vi "0-Do Overlays.vi"(0 "Image Reference\nand Descriptor":cluster{"Image Out":T2, "Image Descriptor":T3} {"Image Descriptor"."Upper-Left Corner Coordinates"."North" format="%#_10f"; "Image Descriptor"."Upper-Left Corner Coordinates"."East" format="%#_8f"}, 1 "Missions":refnum<class "GenericMission.lvclass">[](array[class]), 2 "No Sail Circles":T1[](array[typedef]), 5 "Waypoints":T8, 7 "Current Waypoint #":T7, 9 "Heading":T5 format="%05.1f", 11 "Sail Position":T6=0.5, 12 "Robot UTM Location":T4 {"North" format="%#_10f"; "East" format="%#_8f"}) -> (4 "Image out":T2)   [LabVIEW 2011]
doc: "Overlays waypoints and a boat icon on the image."
uses:
  <vilib>/vision/Image Controls.llb/IMAQ Image.ctl
  0x2-OCU-Think Comm/0x2 Typedefs/Waypoints List.ctl
  2-Think/2 Classes/Waypoint/Waypoint.lvclass
  0x2-OCU-Think Comm/0x2 Typedefs/Current Waypoint.ctl
  2-Think/2 Typedefs/sail setpt.ctl
  2-Think/2 Typedefs/heading.ctl
  2-Think/2 Typedefs/UTM Location.ctl
  0-Image Descriptor.ctl
  2-Think/2 Classes/Missions/GenericMission/GenericMission.lvclass
  2-Think/2 Typedefs/UTM Circle.ctl
panel:
  out "Boat Outside Img":bool
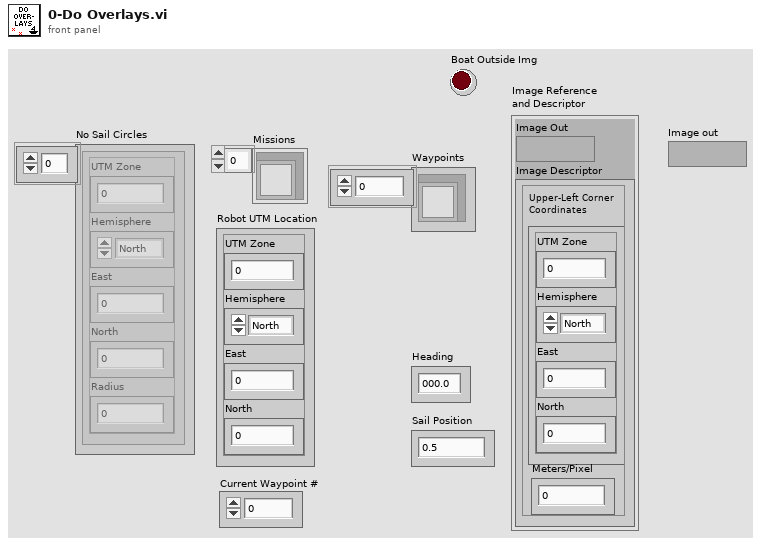
[diagram p1: front panel]
types:
  T1 = typedef "UTM Circle.ctl" = cluster{"UTM Zone":dbl, "Hemisphere":enum16{"North", "South"}, "East":dbl, "North":dbl, "Radius":dbl}
  T2 = typedef "IMAQ Image.ctl" = refnum<image>
  T3 = typedef "0-Image Descriptor.ctl" = cluster{"Upper-Left Corner Coordinates":T4, "Meters/Pixel":dbl}
  T4 = typedef "UTM Location.ctl" = cluster{"UTM Zone":dbl, "Hemisphere":enum16{"North", "South"}, "East":dbl, "North":dbl}
  T5 = typedef "heading.ctl" = dbl
  T6 = typedef "sail setpt.ctl" = dbl
  T7 = typedef "Current Waypoint.ctl" = i32
  T8 = typedef "Waypoints List.ctl" = refnum<class "Waypoint.lvclass">[]
  T9 = typedef "Overlay References.ctl" = cluster{"Boat Icon, Unroatated":T2, "Boat Icon, Rotated":T2, "Sail Icon, Unrotated":T2, "Sail Icon, Rotated":T2}
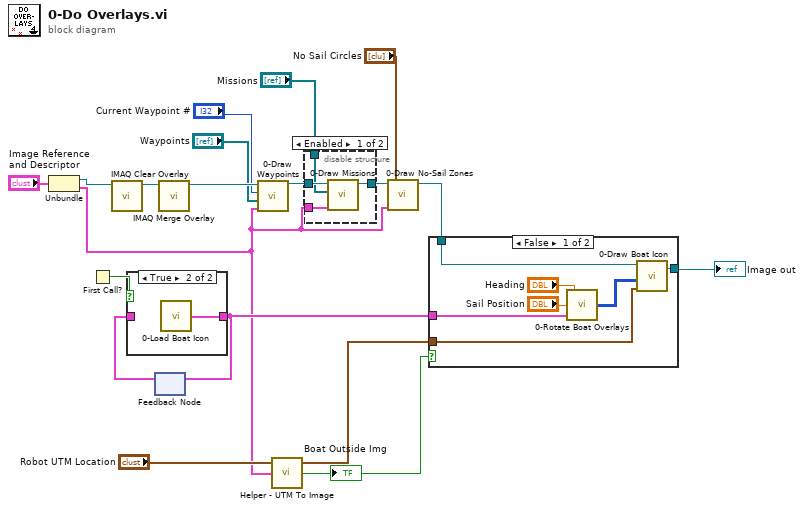
[diagram p0: block diagram]
diagram:
  n1 = Unbundle("Image Reference\nand Descriptor") -> ("Image Out"=w7:T2, "Image Descriptor"=w4:T3)
  n2 = First Call?() -> (First Call?: T/F=w16:bool)
  n3 = call "IMAQ Clear Overlay"("Image"=w7) -> ("Image Out"=w19:T2)  [unwired: 2 in, 8 out]
  n4 = feedback #1() -> (w14:T9)  [unwired: 1 in]
  n5 = case shown="True" w16 {
    tunnel: [w20 w21] -> w15
    tunnel: w14 -> [w20 _]
    frame False {
      # "image already\nloaded"
    }
    frame True {
      n6 = call "0-Load Boat Icon.vi"() -> ("Overlay References Out"=w21:T9)  [unwired: 1 in]
    }
  }
  n7 = feedback-in #1(w15) -> ()
  n8 = call "IMAQ Merge Overlay"("Image Src"=w19) -> ("Image Dst Out"=w17:T2)  [unwired: 4 in, 6 out]
  n9 = call "0-Draw Waypoints.vi"("Image Descriptor"=w4, "Waypoints List"="Waypoints", "Current Waypoint #"="Current Waypoint #", "Image In"=w17) -> ("Image Out"=w6:T2)  [unwired: 2 in, 1 out]
  n10 = call "Helper - UTM To Image.vi"("Image Descriptor"=w4, "UTM Location"="Robot UTM Location") -> ("Coordinate Outside Image"=w11:bool, "Pixel Coordinates"=w10:cluster{"X":i32, "Y":i32})  [unwired: 1 in, 1 out]
  "Boat Outside Img" <- w11
  n11 = disable-structure shown="Enabled" {
    disable-tunnel: w4 -> [w25 _]
    disable-tunnel: w6 -> [w24 w26]
    disable-tunnel: [w23 w26] -> w2
    disable-tunnel: "Missions" -> [w22 _]
    frame Enabled {
      n12 = call "0-Draw Missions.vi"("Image Descriptor"=w25, "Missions"=w22, "Image In"=w24) -> ("Image Out"=w23:T2)  [unwired: 8 in]
    }
    frame Disabled {
    }
  }
  n13 = call "0-Draw No-Sail Zones.vi"("Image Descriptor"=w4, "No Sail Circles"="No Sail Circles", "Image In"=w2) -> ("Image Out"=w3:T2)  [unwired: 3 in, 1 out]
  n14 = case shown="False" w11 {
    tunnel: [w33 w34] -> w18
    tunnel: w3 -> [w32 w34]
    tunnel: w10 -> [w31 _]
    tunnel: w15 -> [w29 _]
    frame False {
      n15 = call "0-Rotate Boat Overlays.vi"("Overlay References In"=w29, "Sail Position"="Sail Position", "Heading"="Heading") -> ("Rotated Boat Icon Bitmap Out"=w30:u32[][])  [unwired: 1 in, 1 out]
      n16 = call "0-Draw Boat Icon.vi"("Position"=w31, "Boat Bitmap"=w30, "Image In"=w32) -> ("Image Out"=w33:T2)  [unwired: 4 out]
    }
    frame True {
      # "don't draw\nif boat\noutside\nimage"
    }
  }
  "Image out" <- w18
